vi "S4GUI_002.vi"(7 "Tab ObsEng":enum32{"Obs", "CCD modes", "Eng"}(tab)) -> ()   [LabVIEW 2018] (continued)
              disable-tunnel: [w7942 w7949] -> w7908
              disable-tunnel: w7907 -> [w7941 w7948]
              disable-tunnel: [w7940 w7948] -> w7906
              frame Disabled {
                n3528 = call-dynamic "Read State Machine.vi"("error in (no error)"=w7941, "Device in"=w7944) -> ("error out"=w7947:errorcluster, "State Machine.lvclass"=w7939:refnum<class "State Machine.lvclass">, "Device out"=w7943:refnum<class "Channel.lvclass">)  [unwired: 7 in]
                n3529 = call "Next State.vi"("error in (no error)"=w7947, "New_State"=12, "State Machine in"=w7939) -> ("error out"=w7946:errorcluster, "State Machine out"=w7938:refnum<class "State Machine.lvclass">)  [unwired: 7 in]
                n3530 = call-dynamic "Write State Machine.vi"("error in (no error)"=w7946, "State Machine.lvclass"=w7938, "Device in"=w7943) -> ("error out"=w7940:errorcluster, "Device out"=w7942:refnum<class "Channel.lvclass">)  [unwired: 7 in]
              }
              frame Enabled {
              }
            }
            n3531 = call-dynamic "Write Channel.vi"("error in (no error)"=w7906, "Channel.lvclass"=w7908, "Acquisition in"=w7922) -> ("error out"=w7920:errorcluster, "Acquisition out"=w7921:refnum<class "Acquisition.lvclass">)  [unwired: 7 in]
            n3532 = call-dynamic "Write AcquisitionD.vi"("error in (no error)"=w7920, "Acquisition.lvclass"=w7921, "S4ACS_GUI in"=w7923) -> ("error out"=w7934:errorcluster, "S4ACS_GUI out"=w7935:refnum<class "S4GUI.lvclass">)  [unwired: 7 in]
          }
        }
      }
      event "Start ch1": Value Change {
        n3533 = event-data() -> ()  [unwired: 1 in, 6 out]
        n3534 = call "Read Instrument.lvclass.vi"("error in (no error)"=w7959, "S4ACS_GUI in"=w7961) -> ("error out"=w7962:errorcluster, "Instrument.lvclass"=w7963:refnum<class "Instrument.lvclass">, "S4ACS_GUI out"=w7960:refnum<class "S4GUI.lvclass">)  [unwired: 7 in]
        n3535 = call-dynamic "Read mode.vi"("error in (no error)"=w7962, "Instrument in"=w7963) -> ("error out"=w7958:errorcluster, "mode"=w7957:bool)  [unwired: 7 in, 1 out]
        n3536 = call-dynamic "Read AcquisitionA.vi"("error in (no error)"=w7958, "S4ACS_GUI in"=w7960) -> ("error out"=w7975:errorcluster, "Acquisition.lvclass"=w7976:refnum<class "Acquisition.lvclass">, "S4ACS_GUI out"=w7978:refnum<class "S4GUI.lvclass">)  [unwired: 7 in]
        n3537 = call-dynamic "Read Acq_state.vi"("error in (no error)"=w7975, "Acquisition in"=w7976) -> ("error out"=w7972:errorcluster, "Acq_state"=w7974:u32, "Acquisition out"=w7971:refnum<class "Acquisition.lvclass">)  [unwired: 7 in]
        n3538 = Not Equal?(x=w7974, y=u32 400) -> (x != y?=w7977:bool)
        n3539 = case shown="True" w7977 {
          tunnel: w7978 -> [w7991 w8030]
          tunnel: [w7991 w8037] -> w7970
          tunnel: [w7986 w8036] -> w7954
          tunnel: w7972 -> [w7993 w8022]
          tunnel: w7971 -> [w7996 w8018]
          tunnel: [w7987 w8010] -> w7969
          tunnel: w7968 -> [_ w8055]
          tunnel: w7967 -> [_ w8054]
          tunnel: w7966 -> [_ w8053]
          tunnel: w7965 -> [_ w8052]
          tunnel: w7964 -> [_ w8047]
          tunnel: w7957 -> [_ w8035]
          tunnel: w7953 -> [_ w8013]
          tunnel: w7952 -> [_ w8016]
          tunnel: w7951 -> [_ w8015]
          tunnel: w7950 -> [_ w8014]
          frame False {
            n3540 = call-dynamic "Read Acq_prevstate.vi"("error in (no error)"=w7993, "Acquisition in"=w7996) -> ("error out"=w7992:errorcluster, "Acq_prevstate"=w7994:u32, "Acquisition out"=w7995:refnum<class "Acquisition.lvclass">)  [unwired: 7 in]
            n3541 = call-dynamic "Write Acq_state.vi"("error in (no error)"=w7992, "Acq_state"=w7994, "Acquisition in"=w7995) -> ("error out"=w7983:errorcluster, "Acquisition out"=w7985:refnum<class "Acquisition.lvclass">)  [unwired: 7 in]
            n3542 = call-dynamic "Read enabled.vi"("error in (no error)"=w7983, "Server in"=w7985) -> ("error out"=w7982:errorcluster, "enabled"=w7979:bool, "Server out"=w7984:refnum<class "Acquisition.lvclass">)  [unwired: 7 in]
            n3543 = call-dynamic "Read Channel.vi"("error in (no error)"=w7982, "Acquisition in"=w7984) -> ("error out"=w7980:errorcluster, "Channel.lvclass"=w7981:refnum<class "Channel.lvclass">, "Acquisition out"=w7990:refnum<class "Acquisition.lvclass">)  [unwired: 7 in]
            n3544 = case shown="True" w7979 {
              tunnel: w7981 -> [w7998 w8008]
              tunnel: [w7998 w8006] -> w7989
              tunnel: w7980 -> [w7997 w8003]
              tunnel: [w7997 w8001] -> w7988
              frame False {
              }
              frame True {
                n3545 = call-dynamic "Read State Machine.vi"("error in (no error)"=w8003, "Device in"=w8008) -> ("error out"=w7999:errorcluster, "State Machine.lvclass"=w8000:refnum<class "State Machine.lvclass">, "Device out"=w8007:refnum<class "Channel.lvclass">)  [unwired: 7 in]
                n3546 = call "Next State.vi"("error in (no error)"=w7999, "New_State"=96, "State Machine in"=w8000) -> ("error out"=w8002:errorcluster, "State Machine out"=w8005:refnum<class "State Machine.lvclass">)  [unwired: 7 in]
                n3547 = call-dynamic "Write State Machine.vi"("error in (no error)"=w8002, "State Machine.lvclass"=w8005, "Device in"=w8007) -> ("error out"=w8001:errorcluster, "Device out"=w8006:refnum<class "Channel.lvclass">)  [unwired: 7 in]
              }
            }
            n3548 = call-dynamic "Write Channel.vi"("error in (no error)"=w7988, "Channel.lvclass"=w7989, "Acquisition in"=w7990) -> ("error out"=w7986:errorcluster, "Acquisition out"=w7987:refnum<class "Acquisition.lvclass">)  [unwired: 7 in]
          }
          frame True {
            # "vide S4GUI:\nHandleObservationAsync.vi"
            # "object"
            # "suffix"
            # "obsType"
            n3549 = call "Read Instrument.lvclass.vi"("S4ACS_GUI in"=w8030) -> ("error out"=w8032:errorcluster, "Instrument.lvclass"=w8034:refnum<class "Instrument.lvclass">, "S4ACS_GUI out"=w8020:refnum<class "S4GUI.lvclass">)  [unwired: 8 in]
            n3550 = call "Read WPROT.vi"("error in (no error)"=w8032, "Instrument in"=w8034) -> ("error out"=w8031:errorcluster, "Opt_Selector.lvclass"=w8033:refnum<class "Opt_Selector.lvclass">)  [unwired: 7 in, 1 out]
            n3551 = call-dynamic "Read sequencia.vi"("error in (no error)"=w8031, "Opt_Selector in"=w8033) -> ("sequencia"=w8029:u16)  [unwired: 7 in, 2 out]
            n3552 = case shown="\"FOCUS\"" w8013 {
              tunnel: [u32 1 ("#cycles ch1") "#cycles ch1"] -> w8038
              tunnel: w8035 -> [_ w8086]
              tunnel: w8029 -> [_ w8085]
              tunnel: [u32 1 w8084] -> w8028
              frame "FOCUS" {
                # "Para sequência de foco, #cycles=1 e #seqs=1."
              }
              frame Default {
                n3553 = case shown="True" w8086 {
                  tunnel: [0 w8090] -> w8084
                  tunnel: w8085 -> [_ w8089]
                  frame False {
                    # "OV 20230424: \n#SEQ agora armazena as\nposições da lâmina utilizadas.\nNa fotometria, #SEQ=0"
                    # "fotometria:"
                  }
                  frame True {
                    # "OV 20230424: \n#SEQ agora armazena as\nposições da lâmina utilizadas.\nNa polarimetria, #SEQ=WPROT.sequencia"
                    # "polarimetria:"
                    n3554 = To Unsigned Long Integer(number=w8089) -> (unsigned 32bit integer=w8090:u32)
                  }
                }
              }
            }
            n3555 = case shown="\"FOCUS\"" w8013 {
              tunnel: [u32 271 ("Obs_state") u32 251 ("Obs_state")] -> w8021
              tunnel: w8022 -> [w8094 w8105]
              tunnel: [w8093 w8105] -> w8017
              tunnel: w8016 -> [w8101 _]
              tunnel: w8015 -> [w8100 _]
              tunnel: w8014 -> [w8099 _]
              tunnel: w8020 -> [w8092 w8104]
              tunnel: [w8091 w8104] -> w8019
              frame "FOCUS" {
                n3556 = call-dynamic "Read TelFocus.lvclass.vi"("error in (no error)"=w8094, "S4GUI in"=w8092) -> ("error out"=w8096:errorcluster, "TelFocus.lvclass"=w8098:refnum<class "TelFocus.lvclass">, "S4GUI out"=w8102:refnum<class "S4GUI.lvclass">)  [unwired: 7 in]
                n3557 = call-dynamic "LoadParam.vi"("#steps"=w8099, "error in (no error)"=w8096, "step"=w8100, "init"=w8101, "TelFocus in"=w8098) -> ("error out"=w8095:errorcluster, "TelFocus out"=w8097:refnum<class "TelFocus.lvclass">)  [unwired: 5 in]
                n3558 = call-dynamic "Write TelFocus.lvclass.vi"("error in (no error)"=w8095, "TelFocus.lvclass"=w8097, "S4GUI in"=w8102) -> ("error out"=w8093:errorcluster, "S4GUI out"=w8091:refnum<class "S4GUI.lvclass">)  [unwired: 7 in]
              }
              frame Default {
              }
            }
            n3559 = property on="Start ch1" class="Bool"(error in=w8022, "DisabledEnum"=T12."Disabled and Grayed Out" ("Disabled")) -> ()  [unwired: 1 in, 2 out]
            n3560 = call-dynamic "Write Acq_state.vi"("error in (no error)"=w8017, "Acq_state"=w8021, "Acquisition in"=w8018) -> ("error out"=w8056:errorcluster, "Acquisition out"=w8057:refnum<class "Acquisition.lvclass">)  [unwired: 7 in]
            n3561 = call-dynamic "Read Channel.vi"("error in (no error)"=w8056, "Acquisition in"=w8057) -> ("error out"=w8058:errorcluster, "Channel.lvclass"=w8059:refnum<class "Channel.lvclass">, "Acquisition out"=w8070:refnum<class "Acquisition.lvclass">)  [unwired: 7 in]
            n3562 = call-dynamic "Read Interface.vi"("error in (no error)"=w8058, "Channel in"=w8059) -> ("error out"=w8080:errorcluster, "Interface.lvclass"=w8081:refnum<class "Interface.lvclass">, "Channel out"=w8079:refnum<class "Channel.lvclass">)  [unwired: 7 in]
            n3563 = call "Write Exposure Time.vi"("error in (no error)"=w8080, "Exposure Time"="Exptime ch1", "Interface in"=w8081) -> ("error out"=w8026:errorcluster, "Interface out"=w8027:refnum<class "Interface.lvclass">)  [unwired: 7 in]
            n3564 = case shown="Default" w8013 {
              tunnel: w8027 -> [w8108 w8113]
              tunnel: w8026 -> [w8107 w8112]
              tunnel: "Exptime ch1" -> [_ w8111]
              tunnel: [w8107 w8110] -> w8024
              tunnel: [w8108 w8109] -> w8023
              frame "ZERO" {
              }
              frame Default {
                n3565 = call-dynamic "Write prev ExpTime.vi"("error in (no error)"=w8112, "prev ExpTime"=w8111, "Interface in"=w8113) -> ("error out"=w8110:errorcluster, "Interface out"=w8109:refnum<class "Interface.lvclass">)  [unwired: 7 in]
              }
            }
            n3566 = call-dynamic "Write Suffix.vi"("error in (no error)"=w8024, "Suffix"=w8055, "Interface in"=w8023) -> ("error out"=w8078:errorcluster, "Interface out"=w8077:refnum<class "Interface.lvclass">)  [unwired: 7 in]
            n3567 = call-dynamic "Write ObsType.vi"("error in (no error)"=w8078, "ObsType"=w8053, "Interface in"=w8077) -> ("error out"=w8075:errorcluster, "Interface out"=w8076:refnum<class "Interface.lvclass">)  [unwired: 7 in]
            n3568 = call-dynamic "Write Object.vi"("error in (no error)"=w8075, "Object"=w8052, "Interface in"=w8076) -> ("error out"=w8074:errorcluster, "Interface out"=w8073:refnum<class "Interface.lvclass">)  [unwired: 7 in]
            n3569 = call-dynamic "Write Comments.vi"("error in (no error)"=w8074, "Comments"=w8054, "Interface in"=w8073) -> ("error out"=w8071:errorcluster, "Interface out"=w8072:refnum<class "Interface.lvclass">)  [unwired: 7 in]
            n3570 = call-dynamic "Write DS9.vi"("error in (no error)"=w8071, "DS9"="F", "Interface in"=w8072) -> ("error out"=w8049:errorcluster, "Interface out"=w8051:refnum<class "Interface.lvclass">)  [unwired: 7 in]
            n3571 = call-dynamic "Write Observer.vi"("error in (no error)"=w8049, "Observer"=w8047, "Interface in"=w8051) -> ("error out"=w8048:errorcluster, "Interface out"=w8050:refnum<class "Interface.lvclass">)  [unwired: 7 in]
            n3572 = call-dynamic "Write # Images.vi"("error in (no error)"=w8048, "# Images"="Exp ch1", "Interface in"=w8050) -> ("error out"=w8067:errorcluster, "Interface out"=w8069:refnum<class "Interface.lvclass">)  [unwired: 7 in]
            n3573 = call-dynamic "Write Interface.vi"("error in (no error)"=w8067, "Interface.lvclass"=w8069, "Channel in"=w8079) -> ("error out"=w8060:errorcluster, "Channel out"=w8061:refnum<class "Channel.lvclass">)  [unwired: 7 in]
            n3574 = property on="Exposure Time ch1" class="Slide (strict)"("Scale.Maximum"="Exptime ch1", "Scale.Minimum"=0.0 ("Scale.Range:Minimum")) -> ()  [unwired: 2 in, 2 out]
            n3575 = property on="Cycles Done ch1" class="Slide (strict)"("Scale.Maximum"=w8038, "Scale.Minimum"=0.0 ("Scale.Range:Minimum")) -> ()  [unwired: 2 in, 2 out]
            n3576 = property on="Exposures Done ch1" class="Slide (strict)"("Scale.Maximum"="Exp ch1", "Scale.Minimum"=0.0 ("Scale.Range:Minimum")) -> ()  [unwired: 2 in, 2 out]
            n3577 = call-dynamic "Write ciclos.vi"("error in (no error)"=w8060, "ciclos"=w8038, "Channel in"=w8061) -> ("error out"=w8045:errorcluster, "Channel out"=w8046:refnum<class "Channel.lvclass">)  [unwired: 7 in]
            n3578 = call-dynamic "Write sequencias.vi"("error in (no error)"=w8045, "sequencias"=w8028, "Channel in"=w8046) -> ("error out"=w8044:errorcluster, "Channel out"=w8043:refnum<class "Channel.lvclass">)  [unwired: 7 in]
            n3579 = call-dynamic "Write Channel.vi"("error in (no error)"=w8044, "Channel.lvclass"=w8043, "Acquisition in"=w8070) -> ("error out"=w8011:errorcluster, "Acquisition out"=w8012:refnum<class "Acquisition.lvclass">)  [unwired: 7 in]
            n3580 = call-dynamic "CalcCubeDuration.vi"("error in (no error)"=w8011, "Acquisition in"=w8012) -> ("error out"=w8009:errorcluster, "Acquisition out"=w8010:refnum<class "Acquisition.lvclass">)  [unwired: 8 in]
            n3581 = call-dynamic "Write sequencias.vi"("error in (no error)"=w8009, "sequencias"=w8028, "S4GUI in"=w8019) -> ("error out"=w8040:errorcluster, "S4GUI out"=w8039:refnum<class "S4GUI.lvclass">)  [unwired: 7 in]
            n3582 = call-dynamic "Write ciclos.vi"("error in (no error)"=w8040, "ciclos"=w8038, "S4ACS_GUI in"=w8039) -> ("error out"=w8041:errorcluster, "S4ACS_GUI out"=w8042:refnum<class "S4GUI.lvclass">)  [unwired: 7 in]
            n3583 = call-dynamic "Write TotalCiclos.vi"("error in (no error)"=w8041, "TotalCiclos"=w8038, "S4GUI in"=w8042) -> ("error out"=w8036:errorcluster, "S4GUI out"=w8037:refnum<class "S4GUI.lvclass">)  [unwired: 7 in]
          }
        }
        n3584 = call-dynamic "Write AcquisitionA.vi"("error in (no error)"=w7954, "Acquisition.lvclass"=w7969, "S4ACS_GUI in"=w7970) -> ("error out"=w7955:errorcluster, "S4ACS_GUI out"=w7956:refnum<class "S4GUI.lvclass">)  [unwired: 7 in]
      }
      event "Start ch2": Value Change {
        n3585 = event-data() -> ()  [unwired: 1 in, 6 out]
        n3586 = call "Read Instrument.lvclass.vi"("error in (no error)"=w8122, "S4ACS_GUI in"=w8123) -> ("error out"=w8124:errorcluster, "Instrument.lvclass"=w8125:refnum<class "Instrument.lvclass">, "S4ACS_GUI out"=w8121:refnum<class "S4GUI.lvclass">)  [unwired: 7 in]
        n3587 = call-dynamic "Read mode.vi"("error in (no error)"=w8124, "Instrument in"=w8125) -> ("error out"=w8120:errorcluster, "mode"=w8119:bool)  [unwired: 7 in, 1 out]
        n3588 = call "Read AcquisitionB.vi"("error in (no error)"=w8120, "S4ACS_GUI in"=w8121) -> ("error out"=w8139:errorcluster, "Acquisition.lvclass"=w8140:refnum<class "Acquisition.lvclass">, "S4ACS_GUI out"=w8142:refnum<class "S4GUI.lvclass">)  [unwired: 7 in]
        n3589 = call-dynamic "Read Acq_state.vi"("error in (no error)"=w8139, "Acquisition in"=w8140) -> ("error out"=w8136:errorcluster, "Acq_state"=w8138:u32, "Acquisition out"=w8135:refnum<class "Acquisition.lvclass">)  [unwired: 7 in]
        n3590 = Not Equal?(x=w8138, y=u32 400) -> (x != y?=w8141:bool)
        n3591 = case shown="True" w8141 {
          tunnel: w8142 -> [w8155 w8195]
          tunnel: [w8155 w8202] -> w8134
          tunnel: [w8150 w8201] -> w8118
          tunnel: w8136 -> [w8157 w8182]
          tunnel: w8135 -> [w8160 w8185]
          tunnel: [w8151 w8173] -> w8133
          tunnel: w8131 -> [_ w8223]
          tunnel: w8130 -> [_ w8222]
          tunnel: w8128 -> [_ w8218]
          tunnel: w8127 -> [_ w8217]
          tunnel: w8126 -> [_ w8211]
          tunnel: w8119 -> [_ w8193]
          tunnel: w8117 -> [_ w8180]
          tunnel: w8116 -> [_ w8179]
          tunnel: w8115 -> [_ w8178]
          tunnel: w8114 -> [_ w8177]
          frame False {
            n3592 = call-dynamic "Read Acq_prevstate.vi"("error in (no error)"=w8157, "Acquisition in"=w8160) -> ("error out"=w8156:errorcluster, "Acq_prevstate"=w8158:u32, "Acquisition out"=w8159:refnum<class "Acquisition.lvclass">)  [unwired: 7 in]
            n3593 = call-dynamic "Write Acq_state.vi"("error in (no error)"=w8156, "Acq_state"=w8158, "Acquisition in"=w8159) -> ("error out"=w8147:errorcluster, "Acquisition out"=w8149:refnum<class "Acquisition.lvclass">)  [unwired: 7 in]
            n3594 = call-dynamic "Read enabled.vi"("error in (no error)"=w8147, "Server in"=w8149) -> ("error out"=w8146:errorcluster, "enabled"=w8143:bool, "Server out"=w8148:refnum<class "Acquisition.lvclass">)  [unwired: 7 in]
            n3595 = call-dynamic "Read Channel.vi"("error in (no error)"=w8146, "Acquisition in"=w8148) -> ("error out"=w8144:errorcluster, "Channel.lvclass"=w8145:refnum<class "Channel.lvclass">, "Acquisition out"=w8154:refnum<class "Acquisition.lvclass">)  [unwired: 7 in]
            n3596 = case shown="True" w8143 {
              tunnel: w8145 -> [w8162 w8172]
              tunnel: [w8162 w8170] -> w8153
              tunnel: w8144 -> [w8161 w8167]
              tunnel: [w8161 w8165] -> w8152
              frame False {
              }
              frame True {
                n3597 = call-dynamic "Read State Machine.vi"("error in (no error)"=w8167, "Device in"=w8172) -> ("error out"=w8163:errorcluster, "State Machine.lvclass"=w8164:refnum<class "State Machine.lvclass">, "Device out"=w8171:refnum<class "Channel.lvclass">)  [unwired: 7 in]
                n3598 = call "Next State.vi"("error in (no error)"=w8163, "New_State"=96, "State Machine in"=w8164) -> ("error out"=w8166:errorcluster, "State Machine out"=w8169:refnum<class "State Machine.lvclass">)  [unwired: 7 in]
                n3599 = call-dynamic "Write State Machine.vi"("error in (no error)"=w8166, "State Machine.lvclass"=w8169, "Device in"=w8171) -> ("error out"=w8165:errorcluster, "Device out"=w8170:refnum<class "Channel.lvclass">)  [unwired: 7 in]
              }
            }
            n3600 = call-dynamic "Write Channel.vi"("error in (no error)"=w8152, "Channel.lvclass"=w8153, "Acquisition in"=w8154) -> ("error out"=w8150:errorcluster, "Acquisition out"=w8151:refnum<class "Acquisition.lvclass">)  [unwired: 7 in]
          }
          frame True {
            # "obs type"
            # "suffix"
            # "object"
            n3601 = call "Read Instrument.lvclass.vi"("S4ACS_GUI in"=w8195) -> ("error out"=w8197:errorcluster, "Instrument.lvclass"=w8199:refnum<class "Instrument.lvclass">, "S4ACS_GUI out"=w8186:refnum<class "S4GUI.lvclass">)  [unwired: 8 in]
            n3602 = call "Read WPROT.vi"("error in (no error)"=w8197, "Instrument in"=w8199) -> ("error out"=w8196:errorcluster, "Opt_Selector.lvclass"=w8198:refnum<class "Opt_Selector.lvclass">)  [unwired: 7 in, 1 out]
            n3603 = call-dynamic "Read sequencia.vi"("error in (no error)"=w8196, "Opt_Selector in"=w8198) -> ("sequencia"=w8192:u16)  [unwired: 7 in, 2 out]
            n3604 = case shown="Default" w8180 {
              tunnel: [u32 1 ("#cycles ch2") "#cycles ch2"] -> w8200
              tunnel: [u32 1 w8253] -> w8194
              tunnel: w8193 -> [_ w8252]
              tunnel: w8192 -> [_ w8251]
              frame "FOCUS" {
              }
              frame Default {
                n3605 = case shown="True" w8252 {
                  tunnel: [0 w8257] -> w8253
                  tunnel: w8251 -> [_ w8256]
                  frame False {
                    # "OV 20230424: \n#SEQ agora armazena as\nposições da lâmina utilizadas.\nNa fotometria, #SEQ=0"
                    # "fotometria:"
                  }
                  frame True {
                    # "OV 20230424: \n#SEQ agora armazena as\nposições da lâmina utilizadas.\nNa polarimetria, #SEQ=WPROT.sequencia"
                    # "polarimetria:"
                    n3606 = To Unsigned Long Integer(number=w8256) -> (unsigned 32bit integer=w8257:u32)
                  }
                }
              }
            }
            n3607 = case shown="Default" w8180 {
              tunnel: [u32 271 ("Obs_state") u32 251 ("Obs_state")] -> w8183
              tunnel: w8182 -> [w8261 w8272]
              tunnel: [w8260 w8272] -> w8181
              tunnel: w8179 -> [w8268 _]
              tunnel: w8178 -> [w8267 _]
              tunnel: w8177 -> [w8266 _]
              tunnel: w8186 -> [w8259 w8271]
              tunnel: [w8258 w8271] -> w8184
              frame "FOCUS" {
                n3608 = call-dynamic "Read TelFocus.lvclass.vi"("error in (no error)"=w8261, "S4GUI in"=w8259) -> ("error out"=w8263:errorcluster, "TelFocus.lvclass"=w8265:refnum<class "TelFocus.lvclass">, "S4GUI out"=w8269:refnum<class "S4GUI.lvclass">)  [unwired: 7 in]
                n3609 = call-dynamic "LoadParam.vi"("#steps"=w8266, "error in (no error)"=w8263, "step"=w8267, "init"=w8268, "TelFocus in"=w8265) -> ("error out"=w8262:errorcluster, "TelFocus out"=w8264:refnum<class "TelFocus.lvclass">)  [unwired: 5 in]
                n3610 = call-dynamic "Write TelFocus.lvclass.vi"("error in (no error)"=w8262, "TelFocus.lvclass"=w8264, "S4GUI in"=w8269) -> ("error out"=w8260:errorcluster, "S4GUI out"=w8258:refnum<class "S4GUI.lvclass">)  [unwired: 7 in]
              }
              frame Default {
              }
            }
            n3611 = property on="Start ch2" class="Bool"(error in=w8182, "DisabledEnum"=T12."Disabled and Grayed Out" ("Disabled")) -> ()  [unwired: 1 in, 2 out]
            n3612 = call-dynamic "Write Acq_state.vi"("error in (no error)"=w8181, "Acq_state"=w8183, "Acquisition in"=w8185) -> ("error out"=w8225:errorcluster, "Acquisition out"=w8226:refnum<class "Acquisition.lvclass">)  [unwired: 7 in]
            n3613 = call-dynamic "Read Channel.vi"("error in (no error)"=w8225, "Acquisition in"=w8226) -> ("error out"=w8227:errorcluster, "Channel.lvclass"=w8228:refnum<class "Channel.lvclass">, "Acquisition out"=w8235:refnum<class "Acquisition.lvclass">)  [unwired: 7 in]
            n3614 = call-dynamic "Read Interface.vi"("error in (no error)"=w8227, "Channel in"=w8228) -> ("error out"=w8247:errorcluster, "Interface.lvclass"=w8248:refnum<class "Interface.lvclass">, "Channel out"=w8246:refnum<class "Channel.lvclass">)  [unwired: 7 in]
            n3615 = call "Write Exposure Time.vi"("error in (no error)"=w8247, "Exposure Time"="Exptime ch2", "Interface in"=w8248) -> ("error out"=w8189:errorcluster, "Interface out"=w8191:refnum<class "Interface.lvclass">)  [unwired: 7 in]
            n3616 = case shown="Default" w8180 {
              tunnel: w8191 -> [w8275 w8280]
              tunnel: [w8275 w8279] -> w8190
              tunnel: w8189 -> [w8274 w8278]
              tunnel: [w8274 w8277] -> w8188
              tunnel: "Exptime ch2" -> [_ w8276]
              frame "ZERO" {
              }
              frame Default {
                n3617 = call-dynamic "Write prev ExpTime.vi"("error in (no error)"=w8278, "prev ExpTime"=w8276, "Interface in"=w8280) -> ("error out"=w8277:errorcluster, "Interface out"=w8279:refnum<class "Interface.lvclass">)  [unwired: 7 in]
              }
            }
            n3618 = call-dynamic "Write # Index.vi"("error in (no error)"=w8188, "# Index"="Index ch2", "Interface in"=w8190) -> ("error out"=w8244:errorcluster, "Interface out"=w8245:refnum<class "Interface.lvclass">)  [unwired: 7 in]
            n3619 = call-dynamic "Write Suffix.vi"("error in (no error)"=w8244, "Suffix"=w8223, "Interface in"=w8245) -> ("error out"=w8243:errorcluster, "Interface out"=w8242:refnum<class "Interface.lvclass">)  [unwired: 7 in]
            n3620 = call-dynamic "Write ObsType.vi"("error in (no error)"=w8243, "ObsType"=w8218, "Interface in"=w8242) -> ("error out"=w8240:errorcluster, "Interface out"=w8241:refnum<class "Interface.lvclass">)  [unwired: 7 in]
            n3621 = call-dynamic "Write Object.vi"("error in (no error)"=w8240, "Object"=w8217, "Interface in"=w8241) -> ("error out"=w8239:errorcluster, "Interface out"=w8238:refnum<class "Interface.lvclass">)  [unwired: 7 in]
            n3622 = call-dynamic "Write Comments.vi"("error in (no error)"=w8239, "Comments"=w8222, "Interface in"=w8238) -> ("error out"=w8236:errorcluster, "Interface out"=w8237:refnum<class "Interface.lvclass">)  [unwired: 7 in]
            n3623 = call-dynamic "Write DS9.vi"("error in (no error)"=w8236, "DS9"="F", "Interface in"=w8237) -> ("error out"=w8214:errorcluster, "Interface out"=w8216:refnum<class "Interface.lvclass">)  [unwired: 7 in]
            n3624 = call-dynamic "Write Observer.vi"("error in (no error)"=w8214, "Observer"=w8211, "Interface in"=w8216) -> ("error out"=w8213:errorcluster, "Interface out"=w8215:refnum<class "Interface.lvclass">)  [unwired: 7 in]
            n3625 = call-dynamic "Write # Images.vi"("error in (no error)"=w8213, "# Images"="Exp ch2", "Interface in"=w8215) -> ("error out"=w8220:errorcluster, "Interface out"=w8219:refnum<class "Interface.lvclass">)  [unwired: 7 in]
            n3626 = property on="Exposure Time ch2" class="Slide (strict)"("Scale.Maximum"="Exptime ch2", "Scale.Minimum"=0.0 ("Scale.Range:Minimum")) -> ()  [unwired: 2 in, 2 out]
            n3627 = call-dynamic "Write Interface.vi"("error in (no error)"=w8220, "Interface.lvclass"=w8219, "Channel in"=w8246) -> ("error out"=w8229:errorcluster, "Channel out"=w8230:refnum<class "Channel.lvclass">)  [unwired: 7 in]
            n3628 = property on="Cycles Done ch2" class="Slide (strict)"("Scale.Maximum"=w8200, "Scale.Minimum"=0.0 ("Scale.Range:Minimum")) -> ()  [unwired: 2 in, 2 out]
            n3629 = property on="Exposures Done ch2" class="Slide (strict)"("Scale.Maximum"="Exp ch2", "Scale.Minimum"=0.0 ("Scale.Range:Minimum")) -> ()  [unwired: 2 in, 2 out]
            n3630 = call-dynamic "Write ciclos.vi"("error in (no error)"=w8229, "ciclos"=w8200, "Channel in"=w8230) -> ("error out"=w8210:errorcluster, "Channel out"=w8209:refnum<class "Channel.lvclass">)  [unwired: 7 in]
            n3631 = call-dynamic "Write sequencias.vi"("error in (no error)"=w8210, "sequencias"=w8194, "Channel in"=w8209) -> ("error out"=w8208:errorcluster, "Channel out"=w8207:refnum<class "Channel.lvclass">)  [unwired: 7 in]
            n3632 = call-dynamic "Write Channel.vi"("error in (no error)"=w8208, "Channel.lvclass"=w8207, "Acquisition in"=w8235) -> ("error out"=w8175:errorcluster, "Acquisition out"=w8176:refnum<class "Acquisition.lvclass">)  [unwired: 7 in]
            n3633 = call-dynamic "CalcCubeDuration.vi"("error in (no error)"=w8175, "Acquisition in"=w8176) -> ("error out"=w8174:errorcluster, "Acquisition out"=w8173:refnum<class "Acquisition.lvclass">)  [unwired: 8 in]
            n3634 = call-dynamic "Write sequencias.vi"("error in (no error)"=w8174, "sequencias"=w8194, "S4GUI in"=w8184) -> ("error out"=w8204:errorcluster, "S4GUI out"=w8203:refnum<class "S4GUI.lvclass">)  [unwired: 7 in]
            n3635 = call-dynamic "Write ciclos.vi"("error in (no error)"=w8204, "ciclos"=w8200, "S4ACS_GUI in"=w8203) -> ("error out"=w8205:errorcluster, "S4ACS_GUI out"=w8206:refnum<class "S4GUI.lvclass">)  [unwired: 7 in]
            n3636 = call-dynamic "Write TotalCiclos.vi"("error in (no error)"=w8205, "TotalCiclos"=w8200, "S4GUI in"=w8206) -> ("error out"=w8201:errorcluster, "S4GUI out"=w8202:refnum<class "S4GUI.lvclass">)  [unwired: 7 in]
          }
        }
        n3637 = call "Write AcquisitionB.vi"("error in (no error)"=w8118, "Acquisition.lvclass"=w8133, "S4ACS_GUI in"=w8134) -> ("error out"=w8132:errorcluster, "S4ACS_GUI out"=w8129:refnum<class "S4GUI.lvclass">)  [unwired: 7 in]
      }
      event "Start ch3": Value Change {
        n3638 = event-data() -> ()  [unwired: 1 in, 6 out]
        n3639 = call "Read Instrument.lvclass.vi"("error in (no error)"=w8288, "S4ACS_GUI in"=w8290) -> ("error out"=w8291:errorcluster, "Instrument.lvclass"=w8292:refnum<class "Instrument.lvclass">, "S4ACS_GUI out"=w8289:refnum<class "S4GUI.lvclass">)  [unwired: 7 in]
        n3640 = call-dynamic "Read mode.vi"("error in (no error)"=w8291, "Instrument in"=w8292) -> ("error out"=w8287:errorcluster, "mode"=w8286:bool)  [unwired: 7 in, 1 out]
        n3641 = call-dynamic "Read AcquisitionC.vi"("error in (no error)"=w8287, "S4ACS_GUI in"=w8289) -> ("error out"=w8306:errorcluster, "Acquisition.lvclass"=w8307:refnum<class "Acquisition.lvclass">, "S4ACS_GUI out"=w8309:refnum<class "S4GUI.lvclass">)  [unwired: 7 in]
        n3642 = call-dynamic "Read Acq_state.vi"("error in (no error)"=w8306, "Acquisition in"=w8307) -> ("error out"=w8303:errorcluster, "Acq_state"=w8305:u32, "Acquisition out"=w8302:refnum<class "Acquisition.lvclass">)  [unwired: 7 in]
        n3643 = Not Equal?(x=w8305, y=u32 400) -> (x != y?=w8308:bool)
        n3644 = case shown="True" w8308 {
          tunnel: w8309 -> [w8322 w8359]
          tunnel: [w8322 w8367] -> w8301
          tunnel: [w8317 w8368] -> w8285
          tunnel: w8303 -> [w8324 w8351]
          tunnel: w8302 -> [w8327 w8352]
          tunnel: [w8318 w8340] -> w8300
          tunnel: w8298 -> [_ w8388]
          tunnel: w8297 -> [_ w8387]
          tunnel: w8295 -> [_ w8383]
          tunnel: w8294 -> [_ w8382]
          tunnel: w8293 -> [_ w8377]
          tunnel: w8286 -> [_ w8364]
          tunnel: w8284 -> [_ w8347]
          tunnel: w8283 -> [_ w8346]
          tunnel: w8282 -> [_ w8345]
          tunnel: w8281 -> [_ w8344]
          frame False {
            n3645 = call-dynamic "Read Acq_prevstate.vi"("error in (no error)"=w8324, "Acquisition in"=w8327) -> ("error out"=w8323:errorcluster, "Acq_prevstate"=w8325:u32, "Acquisition out"=w8326:refnum<class "Acquisition.lvclass">)  [unwired: 7 in]
            n3646 = call-dynamic "Write Acq_state.vi"("error in (no error)"=w8323, "Acq_state"=w8325, "Acquisition in"=w8326) -> ("error out"=w8312:errorcluster, "Acquisition out"=w8314:refnum<class "Acquisition.lvclass">)  [unwired: 7 in]
            n3647 = call-dynamic "Read enabled.vi"("error in (no error)"=w8312, "Server in"=w8314) -> ("error out"=w8311:errorcluster, "enabled"=w8310:bool, "Server out"=w8313:refnum<class "Acquisition.lvclass">)  [unwired: 7 in]
            n3648 = call-dynamic "Read Channel.vi"("error in (no error)"=w8311, "Acquisition in"=w8313) -> ("error out"=w8315:errorcluster, "Channel.lvclass"=w8316:refnum<class "Channel.lvclass">, "Acquisition out"=w8320:refnum<class "Acquisition.lvclass">)  [unwired: 7 in]
            n3649 = case shown="True" w8310 {
              tunnel: w8316 -> [w8329 w8339]
              tunnel: [w8329 w8337] -> w8319
              tunnel: w8315 -> [w8328 w8334]
              tunnel: [w8328 w8332] -> w8321
              frame False {
              }
              frame True {
                n3650 = call-dynamic "Read State Machine.vi"("error in (no error)"=w8334, "Device in"=w8339) -> ("error out"=w8330:errorcluster, "State Machine.lvclass"=w8331:refnum<class "State Machine.lvclass">, "Device out"=w8338:refnum<class "Channel.lvclass">)  [unwired: 7 in]
                n3651 = call "Next State.vi"("error in (no error)"=w8330, "New_State"=96, "State Machine in"=w8331) -> ("error out"=w8333:errorcluster, "State Machine out"=w8336:refnum<class "State Machine.lvclass">)  [unwired: 7 in]
                n3652 = call-dynamic "Write State Machine.vi"("error in (no error)"=w8333, "State Machine.lvclass"=w8336, "Device in"=w8338) -> ("error out"=w8332:errorcluster, "Device out"=w8337:refnum<class "Channel.lvclass">)  [unwired: 7 in]
              }
            }
            n3653 = call-dynamic "Write Channel.vi"("error in (no error)"=w8321, "Channel.lvclass"=w8319, "Acquisition in"=w8320) -> ("error out"=w8317:errorcluster, "Acquisition out"=w8318:refnum<class "Acquisition.lvclass">)  [unwired: 7 in]
          }
          frame True {
            # "obs type"
            # "suffix"
            # "object"
            n3654 = call "Read Instrument.lvclass.vi"("S4ACS_GUI in"=w8359) -> ("error out"=w8361:errorcluster, "Instrument.lvclass"=w8363:refnum<class "Instrument.lvclass">, "S4ACS_GUI out"=w8350:refnum<class "S4GUI.lvclass">)  [unwired: 8 in]
            n3655 = call "Read WPROT.vi"("error in (no error)"=w8361, "Instrument in"=w8363) -> ("error out"=w8360:errorcluster, "Opt_Selector.lvclass"=w8362:refnum<class "Opt_Selector.lvclass">)  [unwired: 7 in, 1 out]
            n3656 = call-dynamic "Read sequencia.vi"("error in (no error)"=w8360, "Opt_Selector in"=w8362) -> ("sequencia"=w8358:u16)  [unwired: 7 in, 2 out]
            n3657 = case shown="\"FOCUS\"" w8347 {
              tunnel: [u32 271 ("Obs_state") u32 251 ("Obs_state")] -> w8348
              tunnel: w8351 -> [w8427 w8438]
              tunnel: [w8426 w8438] -> _
              tunnel: w8346 -> [w8434 _]
              tunnel: w8345 -> [w8433 _]
              tunnel: w8344 -> [w8432 _]
              tunnel: w8350 -> [w8425 w8437]
              tunnel: [w8424 w8437] -> w8349
              frame "FOCUS" {
                n3658 = call-dynamic "Read TelFocus.lvclass.vi"("error in (no error)"=w8427, "S4GUI in"=w8425) -> ("error out"=w8429:errorcluster, "TelFocus.lvclass"=w8431:refnum<class "TelFocus.lvclass">, "S4GUI out"=w8435:refnum<class "S4GUI.lvclass">)  [unwired: 7 in]
                n3659 = call-dynamic "LoadParam.vi"("#steps"=w8432, "error in (no error)"=w8429, "step"=w8433, "init"=w8434, "TelFocus in"=w8431) -> ("error out"=w8428:errorcluster, "TelFocus out"=w8430:refnum<class "TelFocus.lvclass">)  [unwired: 5 in]
                n3660 = call-dynamic "Write TelFocus.lvclass.vi"("error in (no error)"=w8428, "TelFocus.lvclass"=w8430, "S4GUI in"=w8435) -> ("error out"=w8426:errorcluster, "S4GUI out"=w8424:refnum<class "S4GUI.lvclass">)  [unwired: 7 in]
              }
              frame Default {
              }
            }
            n3661 = case shown="Default" w8347 {
              tunnel: [u32 1 ("#cycles ch3") "#cycles ch3"] -> w8366
              tunnel: [u32 1 w8419] -> w8365
              tunnel: w8364 -> [_ w8418]
              tunnel: w8358 -> [_ w8417]
              frame "FOCUS" {
                # "PARA A SEQUÊNCIA DE FOCO, #CYCLES=1 E #SEQS=1"
              }
              frame Default {
                n3662 = case shown="True" w8418 {
                  tunnel: [0 w8423] -> w8419
                  tunnel: w8417 -> [_ w8422]
                  frame False {
                    # "OV 20230424: \n#SEQ agora armazena as\nposições da lâmina utilizadas.\nNa fotometria, #SEQ=0"
                    # "fotometria:"
                  }
                  frame True {
                    # "OV 20230424: \n#SEQ agora armazena as\nposições da lâmina utilizadas.\nNa polarimetria, #SEQ=WPROT.sequencia"
                    # "polarimetria:"
                    n3663 = To Unsigned Long Integer(number=w8422) -> (unsigned 32bit integer=w8423:u32)
                  }
                }
              }
            }
            n3664 = call-dynamic "Write Acq_state.vi"("Acq_state"=w8348, "Acquisition in"=w8352) -> ("error out"=w8390:errorcluster, "Acquisition out"=w8391:refnum<class "Acquisition.lvclass">)  [unwired: 8 in]
            n3665 = call-dynamic "Read Channel.vi"("error in (no error)"=w8390, "Acquisition in"=w8391) -> ("error out"=w8392:errorcluster, "Channel.lvclass"=w8393:refnum<class "Channel.lvclass">, "Acquisition out"=w8401:refnum<class "Acquisition.lvclass">)  [unwired: 7 in]
            n3666 = property on="Start ch3" class="Bool"(error in=w8351, "DisabledEnum"=T12."Disabled and Grayed Out" ("Disabled")) -> ()  [unwired: 1 in, 2 out]
            n3667 = call-dynamic "Read Interface.vi"("error in (no error)"=w8392, "Channel in"=w8393) -> ("error out"=w8413:errorcluster, "Interface.lvclass"=w8414:refnum<class "Interface.lvclass">, "Channel out"=w8412:refnum<class "Channel.lvclass">)  [unwired: 7 in]
            n3668 = call "Write Exposure Time.vi"("error in (no error)"=w8413, "Exposure Time"="Exptime ch3", "Interface in"=w8414) -> ("error out"=w8355:errorcluster, "Interface out"=w8356:refnum<class "Interface.lvclass">)  [unwired: 7 in]
            n3669 = case shown="\"ZERO\"" w8347 {
              tunnel: [w8440 w8446] -> w8357
              tunnel: w8356 -> [w8440 w8445]
              tunnel: w8355 -> [w8441 w8444]
              tunnel: [w8441 w8443] -> w8354
              tunnel: "Exptime ch3" -> [_ w8442]
              frame "ZERO" {
              }
              frame Default {
                n3670 = call-dynamic "Write prev ExpTime.vi"("error in (no error)"=w8444, "prev ExpTime"=w8442, "Interface in"=w8445) -> ("error out"=w8443:errorcluster, "Interface out"=w8446:refnum<class "Interface.lvclass">)  [unwired: 7 in]
              }
            }
            n3671 = call-dynamic "Write # Index.vi"("error in (no error)"=w8354, "# Index"="Index ch3", "Interface in"=w8357) -> ("error out"=w8410:errorcluster, "Interface out"=w8411:refnum<class "Interface.lvclass">)  [unwired: 7 in]
            n3672 = call-dynamic "Write Suffix.vi"("error in (no error)"=w8410, "Suffix"=w8388, "Interface in"=w8411) -> ("error out"=w8409:errorcluster, "Interface out"=w8408:refnum<class "Interface.lvclass">)  [unwired: 7 in]
            n3673 = call-dynamic "Write ObsType.vi"("error in (no error)"=w8409, "ObsType"=w8382, "Interface in"=w8408) -> ("error out"=w8406:errorcluster, "Interface out"=w8407:refnum<class "Interface.lvclass">)  [unwired: 7 in]
            n3674 = call-dynamic "Write Object.vi"("error in (no error)"=w8406, "Object"=w8383, "Interface in"=w8407) -> ("error out"=w8405:errorcluster, "Interface out"=w8404:refnum<class "Interface.lvclass">)  [unwired: 7 in]
            n3675 = call-dynamic "Write Comments.vi"("error in (no error)"=w8405, "Comments"=w8387, "Interface in"=w8404) -> ("error out"=w8402:errorcluster, "Interface out"=w8403:refnum<class "Interface.lvclass">)  [unwired: 7 in]
            n3676 = call-dynamic "Write DS9.vi"("error in (no error)"=w8402, "DS9"="F", "Interface in"=w8403) -> ("error out"=w8379:errorcluster, "Interface out"=w8381:refnum<class "Interface.lvclass">)  [unwired: 7 in]
            n3677 = call-dynamic "Write Observer.vi"("error in (no error)"=w8379, "Observer"=w8377, "Interface in"=w8381) -> ("error out"=w8378:errorcluster, "Interface out"=w8380:refnum<class "Interface.lvclass">)  [unwired: 7 in]
            n3678 = call-dynamic "Write # Images.vi"("error in (no error)"=w8378, "# Images"="Exp ch3", "Interface in"=w8380) -> ("error out"=w8384:errorcluster, "Interface out"=w8385:refnum<class "Interface.lvclass">)  [unwired: 7 in]
            n3679 = call-dynamic "Write Interface.vi"("error in (no error)"=w8384, "Interface.lvclass"=w8385, "Channel in"=w8412) -> ("error out"=w8394:errorcluster, "Channel out"=w8395:refnum<class "Channel.lvclass">)  [unwired: 7 in]
            n3680 = property on="Exposure Time ch3" class="Slide (strict)"("Scale.Maximum"="Exptime ch3", "Scale.Minimum"=0.0 ("Scale.Range:Minimum")) -> ()  [unwired: 2 in, 2 out]
            n3681 = property on="Exposures Done ch3" class="Slide (strict)"("Scale.Maximum"="Exp ch3", "Scale.Minimum"=0.0 ("Scale.Range:Minimum")) -> ()  [unwired: 2 in, 2 out]
            n3682 = property on="Cycles Done ch3" class="Slide (strict)"("Scale.Maximum"=w8366, "Scale.Minimum"=0.0 ("Scale.Range:Minimum")) -> ()  [unwired: 2 in, 2 out]
            n3683 = call-dynamic "Write ciclos.vi"("error in (no error)"=w8394, "ciclos"=w8366, "Channel in"=w8395) -> ("error out"=w8375:errorcluster, "Channel out"=w8376:refnum<class "Channel.lvclass">)  [unwired: 7 in]
            n3684 = call-dynamic "Write sequencias.vi"("error in (no error)"=w8375, "sequencias"=w8365, "Channel in"=w8376) -> ("error out"=w8373:errorcluster, "Channel out"=w8374:refnum<class "Channel.lvclass">)  [unwired: 7 in]
            n3685 = call-dynamic "Write Channel.vi"("error in (no error)"=w8373, "Channel.lvclass"=w8374, "Acquisition in"=w8401) -> ("error out"=w8342:errorcluster, "Acquisition out"=w8343:refnum<class "Acquisition.lvclass">)  [unwired: 7 in]
            n3686 = call-dynamic "CalcCubeDuration.vi"("error in (no error)"=w8342, "Acquisition in"=w8343) -> ("error out"=w8341:errorcluster, "Acquisition out"=w8340:refnum<class "Acquisition.lvclass">)  [unwired: 8 in]
            n3687 = call-dynamic "Write sequencias.vi"("error in (no error)"=w8341, "sequencias"=w8365, "S4GUI in"=w8349) -> ("error out"=w8370:errorcluster, "S4GUI out"=w8369:refnum<class "S4GUI.lvclass">)  [unwired: 7 in]
            n3688 = call-dynamic "Write ciclos.vi"("error in (no error)"=w8370, "ciclos"=w8366, "S4ACS_GUI in"=w8369) -> ("error out"=w8371:errorcluster, "S4ACS_GUI out"=w8372:refnum<class "S4GUI.lvclass">)  [unwired: 7 in]
            n3689 = call-dynamic "Write TotalCiclos.vi"("error in (no error)"=w8371, "TotalCiclos"=w8366, "S4GUI in"=w8372) -> ("error out"=w8368:errorcluster, "S4GUI out"=w8367:refnum<class "S4GUI.lvclass">)  [unwired: 7 in]
          }
        }
        n3690 = call-dynamic "Write AcquisitionC.vi"("error in (no error)"=w8285, "Acquisition.lvclass"=w8300, "S4ACS_GUI in"=w8301) -> ("error out"=w8299:errorcluster, "S4ACS_GUI out"=w8296:refnum<class "S4GUI.lvclass">)  [unwired: 7 in]
      }
      event "Start ch4": Value Change {
        n3691 = event-data() -> ()  [unwired: 1 in, 6 out]
        n3692 = call "Read Instrument.lvclass.vi"("error in (no error)"=w8456, "S4ACS_GUI in"=w8457) -> ("error out"=w8458:errorcluster, "Instrument.lvclass"=w8459:refnum<class "Instrument.lvclass">, "S4ACS_GUI out"=w8455:refnum<class "S4GUI.lvclass">)  [unwired: 7 in]
        n3693 = call-dynamic "Read mode.vi"("error in (no error)"=w8458, "Instrument in"=w8459) -> ("error out"=w8454:errorcluster, "mode"=w8453:bool)  [unwired: 7 in, 1 out]
        n3694 = call-dynamic "Read AcquisitionD.vi"("error in (no error)"=w8454, "S4ACS_GUI in"=w8455) -> ("error out"=w8472:errorcluster, "Acquisition.lvclass"=w8473:refnum<class "Acquisition.lvclass">, "S4ACS_GUI out"=w8475:refnum<class "S4GUI.lvclass">)  [unwired: 7 in]
        n3695 = call-dynamic "Read Acq_state.vi"("error in (no error)"=w8472, "Acquisition in"=w8473) -> ("error out"=w8469:errorcluster, "Acq_state"=w8471:u32, "Acquisition out"=w8468:refnum<class "Acquisition.lvclass">)  [unwired: 7 in]
        n3696 = Not Equal?(x=w8471, y=u32 400) -> (x != y?=w8474:bool)
        n3697 = case shown="False" w8474 {
          tunnel: w8475 -> [w8488 w8526]
          tunnel: [w8484 w8534] -> w8452
          tunnel: w8469 -> [w8490 w8517]
          tunnel: w8468 -> [w8493 w8518]
          tunnel: [w8483 w8506] -> w8467
          tunnel: w8465 -> [_ w8555]
          tunnel: w8464 -> [_ w8554]
          tunnel: w8462 -> [_ w8550]
          tunnel: w8461 -> [_ w8549]
          tunnel: w8460 -> [_ w8544]
          tunnel: w8453 -> [_ w8532]
          tunnel: [w8488 w8535] -> w8451
          tunnel: w8450 -> [_ w8513]
          tunnel: w8449 -> [_ w8512]
          tunnel: w8448 -> [_ w8511]
          tunnel: w8447 -> [_ w8510]
          frame False {
            n3698 = call-dynamic "Read Acq_prevstate.vi"("error in (no error)"=w8490, "Acquisition in"=w8493) -> ("error out"=w8489:errorcluster, "Acq_prevstate"=w8491:u32, "Acquisition out"=w8492:refnum<class "Acquisition.lvclass">)  [unwired: 7 in]
            n3699 = call-dynamic "Write Acq_state.vi"("error in (no error)"=w8489, "Acq_state"=w8491, "Acquisition in"=w8492) -> ("error out"=w8478:errorcluster, "Acquisition out"=w8482:refnum<class "Acquisition.lvclass">)  [unwired: 7 in]
            n3700 = call-dynamic "Read enabled.vi"("error in (no error)"=w8478, "Server in"=w8482) -> ("error out"=w8477:errorcluster, "enabled"=w8476:bool, "Server out"=w8481:refnum<class "Acquisition.lvclass">)  [unwired: 7 in]
            n3701 = call-dynamic "Read Channel.vi"("error in (no error)"=w8477, "Acquisition in"=w8481) -> ("error out"=w8479:errorcluster, "Channel.lvclass"=w8480:refnum<class "Channel.lvclass">, "Acquisition out"=w8486:refnum<class "Acquisition.lvclass">)  [unwired: 7 in]
            n3702 = case shown="True" w8476 {
              tunnel: w8480 -> [w8495 w8505]
              tunnel: [w8495 w8503] -> w8485
              tunnel: w8479 -> [w8494 w8500]
              tunnel: [w8494 w8498] -> w8487
              frame False {
              }
              frame True {
                n3703 = call-dynamic "Read State Machine.vi"("error in (no error)"=w8500, "Device in"=w8505) -> ("error out"=w8496:errorcluster, "State Machine.lvclass"=w8497:refnum<class "State Machine.lvclass">, "Device out"=w8504:refnum<class "Channel.lvclass">)  [unwired: 7 in]
                n3704 = call "Next State.vi"("error in (no error)"=w8496, "New_State"=96, "State Machine in"=w8497) -> ("error out"=w8499:errorcluster, "State Machine out"=w8502:refnum<class "State Machine.lvclass">)  [unwired: 7 in]
                n3705 = call-dynamic "Write State Machine.vi"("error in (no error)"=w8499, "State Machine.lvclass"=w8502, "Device in"=w8504) -> ("error out"=w8498:errorcluster, "Device out"=w8503:refnum<class "Channel.lvclass">)  [unwired: 7 in]
              }
            }
            n3706 = call-dynamic "Write Channel.vi"("error in (no error)"=w8487, "Channel.lvclass"=w8485, "Acquisition in"=w8486) -> ("error out"=w8484:errorcluster, "Acquisition out"=w8483:refnum<class "Acquisition.lvclass">)  [unwired: 7 in]
          }
          frame True {
            # "obs type"
            # "suffix"
            # "object"
            n3707 = call "Read Instrument.lvclass.vi"("S4ACS_GUI in"=w8526) -> ("error out"=w8528:errorcluster, "Instrument.lvclass"=w8530:refnum<class "Instrument.lvclass">, "S4ACS_GUI out"=w8515:refnum<class "S4GUI.lvclass">)  [unwired: 8 in]
            n3708 = call "Read WPROT.vi"("error in (no error)"=w8528, "Instrument in"=w8530) -> ("error out"=w8527:errorcluster, "Opt_Selector.lvclass"=w8529:refnum<class "Opt_Selector.lvclass">)  [unwired: 7 in, 1 out]
            n3709 = call-dynamic "Read sequencia.vi"("error in (no error)"=w8527, "Opt_Selector in"=w8529) -> ("sequencia"=w8525:u16)  [unwired: 7 in, 2 out]
            n3710 = case shown="\"FOCUS\"" w8513 {
              tunnel: [u32 271 ("Obs_state") u32 251 ("Obs_state")] -> w8519
              tunnel: w8517 -> [w8594 w8605]
              tunnel: [w8593 w8605] -> w8516
              tunnel: w8512 -> [w8601 _]
              tunnel: w8511 -> [w8600 _]
              tunnel: w8510 -> [w8599 _]
              tunnel: w8515 -> [w8592 w8604]
              tunnel: [w8591 w8604] -> w8514
              frame "FOCUS" {
                n3711 = call-dynamic "Read TelFocus.lvclass.vi"("error in (no error)"=w8594, "S4GUI in"=w8592) -> ("error out"=w8596:errorcluster, "TelFocus.lvclass"=w8598:refnum<class "TelFocus.lvclass">, "S4GUI out"=w8602:refnum<class "S4GUI.lvclass">)  [unwired: 7 in]
                n3712 = call-dynamic "LoadParam.vi"("#steps"=w8599, "error in (no error)"=w8596, "step"=w8600, "init"=w8601, "TelFocus in"=w8598) -> ("error out"=w8595:errorcluster, "TelFocus out"=w8597:refnum<class "TelFocus.lvclass">)  [unwired: 5 in]
                n3713 = call-dynamic "Write TelFocus.lvclass.vi"("error in (no error)"=w8595, "TelFocus.lvclass"=w8597, "S4GUI in"=w8602) -> ("error out"=w8593:errorcluster, "S4GUI out"=w8591:refnum<class "S4GUI.lvclass">)  [unwired: 7 in]
              }
              frame Default {
              }
            }
            n3714 = case shown="\"FOCUS\"" w8513 {
              tunnel: [u32 1 ("#cycles ch4") "#cycles ch4"] -> w8533
              tunnel: w8532 -> [_ w8586]
              tunnel: [u32 1 w8585] -> w8531
              tunnel: w8525 -> [_ w8584]
              frame "FOCUS" {
                # "Na sequência de foco, #cycles=1 e #seqs=1"
              }
              frame Default {
                n3715 = case shown="True" w8586 {
                  tunnel: [0 w8590] -> w8585
                  tunnel: w8584 -> [_ w8589]
                  frame False {
                    # "OV 20230424: \n#SEQ agora armazena as\nposições da lâmina utilizadas.\nNa fotometria, #SEQ=0"
                    # "fotometria:"
                  }
                  frame True {
                    # "OV 20230424: \n#SEQ agora armazena as\nposições da lâmina utilizadas.\nNa polarimetria, #SEQ=WPROT.sequencia"
                    # "polarimetria:"
                    n3716 = To Unsigned Long Integer(number=w8589) -> (unsigned 32bit integer=w8590:u32)
                  }
                }
              }
            }
            n3717 = call-dynamic "Write Acq_state.vi"("error in (no error)"=w8516, "Acq_state"=w8519, "Acquisition in"=w8518) -> ("error out"=w8557:errorcluster, "Acquisition out"=w8558:refnum<class "Acquisition.lvclass">)  [unwired: 7 in]
            n3718 = call-dynamic "Read Channel.vi"("error in (no error)"=w8557, "Acquisition in"=w8558) -> ("error out"=w8559:errorcluster, "Channel.lvclass"=w8560:refnum<class "Channel.lvclass">, "Acquisition out"=w8568:refnum<class "Acquisition.lvclass">)  [unwired: 7 in]
            n3719 = call-dynamic "Read Interface.vi"("error in (no error)"=w8559, "Channel in"=w8560) -> ("error out"=w8580:errorcluster, "Interface.lvclass"=w8581:refnum<class "Interface.lvclass">, "Channel out"=w8579:refnum<class "Channel.lvclass">)  [unwired: 7 in]
            n3720 = property on="Start ch4" class="Bool"(error in=w8517, "DisabledEnum"=T12."Disabled and Grayed Out" ("Disabled")) -> ()  [unwired: 1 in, 2 out]
            n3721 = call "Write Exposure Time.vi"("error in (no error)"=w8580, "Exposure Time"="Exptime ch4", "Interface in"=w8581) -> ("error out"=w8521:errorcluster, "Interface out"=w8524:refnum<class "Interface.lvclass">)  [unwired: 7 in]
            n3722 = case shown="\"ZERO\"" w8513 {
              tunnel: w8524 -> [w8608 w8613]
              tunnel: [w8608 w8612] -> w8523
              tunnel: [w8607 w8611] -> w8522
              tunnel: w8521 -> [w8607 w8610]
              tunnel: "Exptime ch4" -> [_ w8609]
              frame "ZERO" {
              }
              frame Default {
                n3723 = call-dynamic "Write prev ExpTime.vi"("error in (no error)"=w8610, "prev ExpTime"=w8609, "Interface in"=w8613) -> ("error out"=w8611:errorcluster, "Interface out"=w8612:refnum<class "Interface.lvclass">)  [unwired: 7 in]
              }
            }
            n3724 = call-dynamic "Write # Index.vi"("error in (no error)"=w8522, "# Index"="Index ch4", "Interface in"=w8523) -> ("error out"=w8577:errorcluster, "Interface out"=w8578:refnum<class "Interface.lvclass">)  [unwired: 7 in]
            n3725 = call-dynamic "Write Suffix.vi"("error in (no error)"=w8577, "Suffix"=w8555, "Interface in"=w8578) -> ("error out"=w8576:errorcluster, "Interface out"=w8575:refnum<class "Interface.lvclass">)  [unwired: 7 in]
            n3726 = call-dynamic "Write ObsType.vi"("error in (no error)"=w8576, "ObsType"=w8550, "Interface in"=w8575) -> ("error out"=w8573:errorcluster, "Interface out"=w8574:refnum<class "Interface.lvclass">)  [unwired: 7 in]
            n3727 = call-dynamic "Write Object.vi"("error in (no error)"=w8573, "Object"=w8549, "Interface in"=w8574) -> ("error out"=w8572:errorcluster, "Interface out"=w8571:refnum<class "Interface.lvclass">)  [unwired: 7 in]
            n3728 = call-dynamic "Write Comments.vi"("error in (no error)"=w8572, "Comments"=w8554, "Interface in"=w8571) -> ("error out"=w8569:errorcluster, "Interface out"=w8570:refnum<class "Interface.lvclass">)  [unwired: 7 in]
            n3729 = call-dynamic "Write DS9.vi"("error in (no error)"=w8569, "DS9"="F", "Interface in"=w8570) -> ("error out"=w8546:errorcluster, "Interface out"=w8548:refnum<class "Interface.lvclass">)  [unwired: 7 in]
